vi "Find Installs.vi"(8 "error in":errorcluster, 11 "ITSDiscovery in":refnum<class "ITSDiscovery.lvclass">) -> (0 "error out":errorcluster, 3 "TSInstalls Out":T1[](array[typedef]))   [LabVIEW 2025, in "ITSDiscovery.lvclass"]
doc: "FindInstalls.vi discovers all NI TestStand installations available on the current system and returns them as an array of TSInstall elements. This abstract implementation only defines inputs and outputs."
uses:
  ITSDiscovery.lvclass
  Type Definitions/TSInstall--cluster.ctl
  Type Definitions/Architecture--enum.ctl
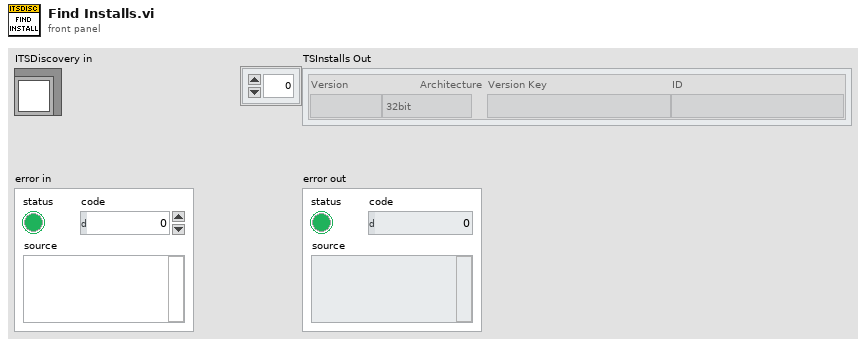
[diagram p1: front panel]
types:
  T1 = typedef "TSInstall--cluster.ctl" = cluster{"Version":string, "Architecture":T2, "Version Key":string, "ID":string}
  T2 = typedef "Architecture--enum.ctl" = enum16{"32bit", "64bit"}
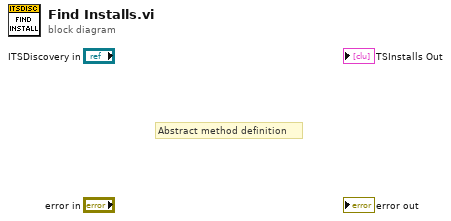
[diagram p0: block diagram]
diagram:
  # "Abstract method definition"
